vi "ble_write_by_handle_uint16.vi"(6 "Connection Status":T1={"MAC Address"="", "cnx handle"=0, "cnx flags"=0, "Address Type"=125, "Connection Interval (ms)"=125, "Timeout(ms)"=125, "Latency"=0, "bonding handle"=0} {"Address Type" items=["Public", "Random"]}, 7 "Handle":u16=1 format="%04x", 8 "error in (no error)":errorcluster, 10 "Value(uint16)":u16 format="%04x", 11 "COM Bluegiga in":refnum<visa-resource-name>) -> (0 "error out":errorcluster, 3 "COM Bluegiga out":refnum<visa-resource-name>)   [LabVIEW 2015]
uses:
  type_def/connection_status_bundle.ctl
  type_def/address_type.ctl
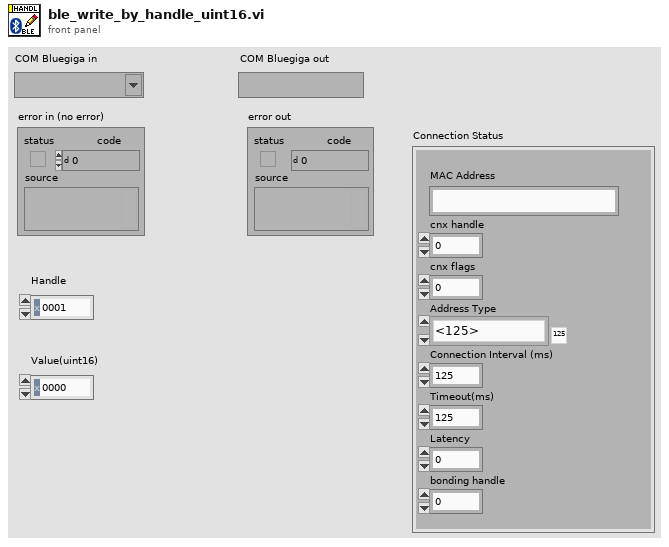
[diagram p1: front panel]
types:
  T1 = typedef "connection_status_bundle.ctl" = cluster{"MAC Address":string, "cnx handle":u8, "cnx flags":u8, "Address Type":T2, "Connection Interval (ms)":u16, "Timeout(ms)":u16, "Latency":u16, "bonding handle":u8}
  T2 = typedef "address_type.ctl" = u8
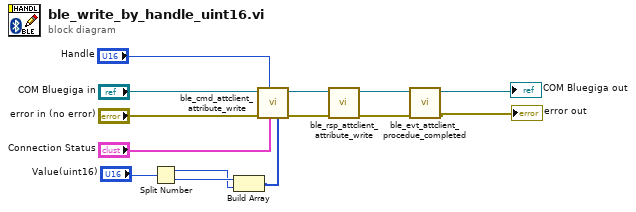
[diagram p0: block diagram]
diagram:
  n1 = Split Number(x="Value(uint16)") -> (hi(x)=w1:u8, lo(x)=w3:u8)
  n2 = Build Array(w3, w1) -> (w2:u8[])
  n3 = call "ble_cmd_attclient_attribute_write.vi"("data (uint8array)"=w2, "Connection Status"="Connection Status", "chrHandle"="Handle", "error in (no error)"="error in (no error)", "COM Bluegiga in"="COM Bluegiga in") -> ("error out"=w11:errorcluster, "COM Bluegiga out"=w12:refnum<visa-resource-name>)  [unwired: 5 in]
  n4 = call "ble_rsp_attclient_attribute_write.vi"("error in (no error)"=w11, "COM Bluegiga in"=w12) -> ("error out"=w9:errorcluster, "COM Bluegiga out"=w10:refnum<visa-resource-name>)  [unwired: 6 in, 2 out]
  n5 = call "ble_evt_attclient_procedue_completed.vi"("error in (no error)"=w9, "COM Bluegiga in"=w10) -> ("error out"=→"error out":errorcluster, "COM Bluegiga out"=→"COM Bluegiga out":refnum<visa-resource-name>)  [unwired: 8 in]
